vi "M14_IR&Limits_Hardware_Globals.vi"() -> ()   [LabVIEW 2019]
panel:
  in  "Beam_Break_B":string="Beam_Break_B"
  in  "Beam_Break_A":string="Beam_Break_A"
  in  "Climber_Limit_B":string="Climber_Limit_B"
  in  "Climber_Limit_A":string="Climber_Limit_A"
  in  "IR_10-oclock":string="IR_10-oclock"
  in  "IR_8-oclock":string="IR_8-oclock"
  in  "IR_5-oclock":string="IR_5-oclock"
  in  "IR_3-oclock":string="IR_3-oclock"
  in  "IR_12-oclock":string="IR_12-oclock"
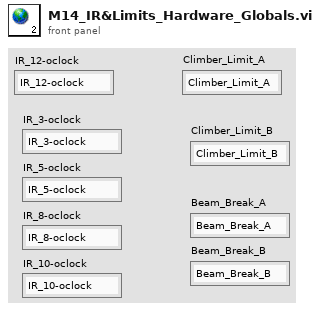
[diagram p1: front panel]
diagram:
